vi "Datasheet Retrieve Table Data.vi"(4 "Datasheets to Generate":T3[](array[typedef]), 5 "Grouped Results":cluster{"Result Group":T6[]}[](array[cluster]), 6 "Paths":T5[](array[typedef]), 7 "Generator Settings":T2={"Wait? (t)"=TRUE, "ClientPrint? (f)"=FALSE, "Client (\"\")"="", "joinPDF"=FALSE, "Sort Method"=enum."Item", "Export Row (-1=all)"=-1, "Preview"=FALSE, "Estimate Time"=FALSE, "username"="", "jobid"=""}, 8 "error in (no error)":errorcluster, 9 "Parameters":T4, 10 "Template Record":T7, 11 "Connection Refnum":T1) -> (0 "error out":errorcluster, 1 "Datasheets to Generate":T3[](array[typedef]), 2 "Paths":T5[](array[typedef]), 3 "Connection Refnum":T1)   [LabVIEW 2011]
uses:
  database/Templates/Template Record.ctl
  Addons/internet/utils/keyedarr.llb/Keyed Array.ctl
  www/cgi-bin/_cgi-lib/TDM_INDEX Record.ctl
  SI.LIB/ODBC/SQL Controls/Connection Refnum.ctl
  Datasheet Report Info.ctl
  lib/datasheet script data.ctl
  Datasheet Generator Settings.ctl
  Addons/internet/utils/strutil.llb/Case Matching.ctl
  Column Data.ctl
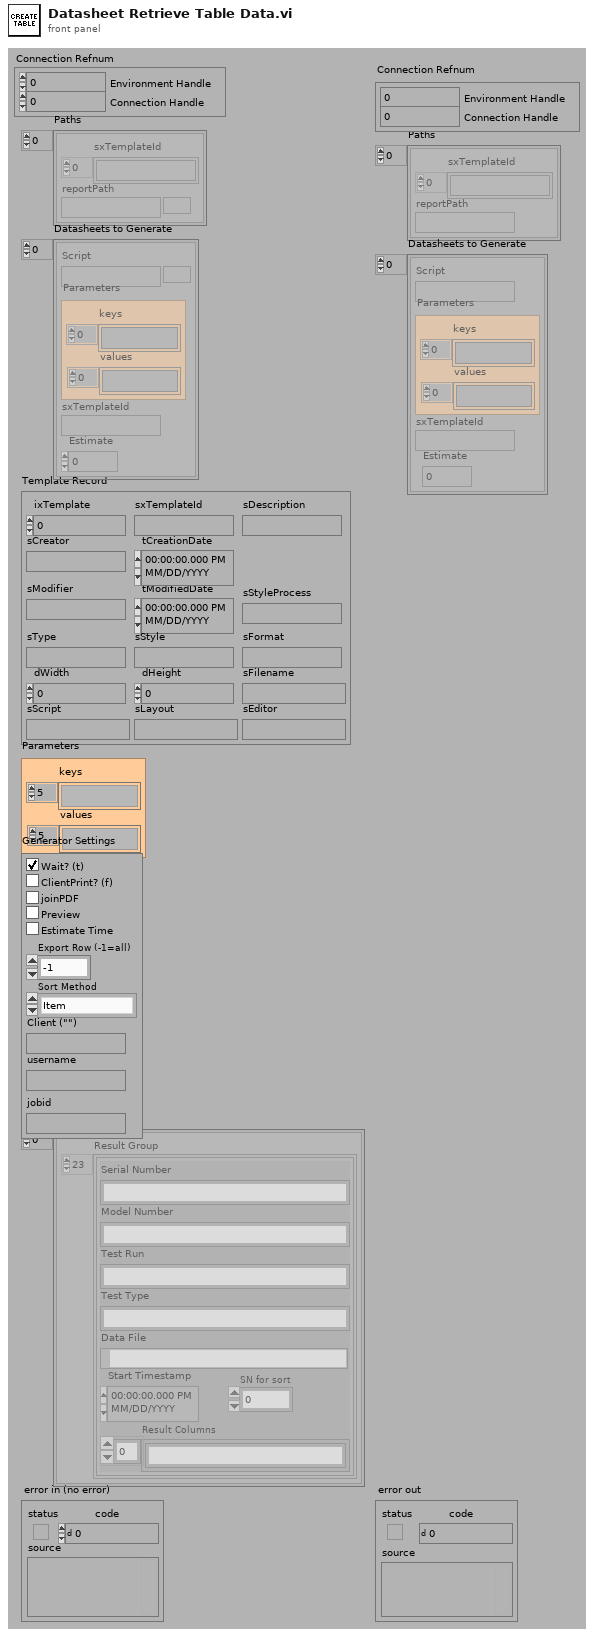
[diagram p1: front panel]
types:
  T1 = typedef "Connection Refnum.ctl" = cluster{"Environment Handle":i32, "Connection Handle":i32}
  T2 = typedef "DATASHEET Generator Settings.ctl" = cluster{"Wait? (t)":bool, "ClientPrint? (f)":bool, "Client (\"\")":string, "joinPDF":bool, "Sort Method":enum16{"Item", "Template", "No Sort"}, "Export Row (-1=all)":i32, "Preview":bool, "Estimate Time":bool, "username":string, "jobid":string}
  T3 = typedef "datasheet script data.ctl" = cluster{"Script":path, "Parameters":T4, "sxTemplateId":string, "Estimate":i32}
  T4 = typedef "Keyed Array.ctl" = cluster{"keys":string[], "values":string[]}
  T5 = typedef "Datasheet Report Info.ctl" = cluster{"sxTemplateId":string[], "reportPath":path}
  T6 = typedef "TDM_INDEX Record.ctl" = cluster{"Model Number":string, "SN for sort":i32, "Test Type":string, "Test Run":string, "Serial Number":string, "Start Timestamp":timestamp, "Data File":path, "Result Columns":string[]}
  T7 = typedef "Template Record.ctl" = cluster{"ixTemplate":i32, "sxTemplateId":string, "sDescription":string, "sCreator":string, "tCreationDate":timestamp, "sModifier":string, "tModifiedDate":timestamp, "sType":string, "sStyle":string, "sFormat":string, "dWidth":dbl, "dHeight":dbl, "sFilename":string, "sScript":string, "sLayout":string, "sEditor":string, "sStyleProcess":string}
  T8 = typedef "Case Matching.ctl" = enum16{"a != A", "a == A", "system"}
  T9 = typedef "Column Data.ctl" = cluster{"Run Select (Field=value)":string, "Type":string, "Parameters (comma list)":string, "Column Label":string}
  T10 = typedef "Field Record.ctl" = cluster{"ixField":i32, "iSequenceOrder":i32, "sxFieldId":string, "sxSequenceId":string, "sDisplayName":string, "sValue":string, "sUnits":string, "nDataType":T11, "nNextItem":T12, "fSystem":bool, "fSystemValue":bool, "fRequired":bool, "fSetAtTest":bool, "fTestField":bool, "fDeleted":bool, "fIndexed":bool, "fFreeList":bool}
  T11 = typedef "Field DataTypes.ctl" = enum32{"text", "numeric", "list", "timestamp", "boolean"}
  T12 = typedef "Field NextItem.ctl" = enum32{"Reset", "Retain", "Auto-Increment"}
  T13 = typedef "TDMS Model Number.ctl" = cluster{"Model Number":string, "Serial Number Tree Data":T14[]}
  T14 = typedef "TDMS Serial Number.ctl" = cluster{"Serial Number":string, "TDM Files":T15[]}
  T15 = typedef "TDMS File.ctl" = cluster{"File Path":path, "Run Data":T16[], "Serial Number":string, "Model Number":string, "Test Type":string}
  T16 = typedef "TDMS Run.ctl" = cluster{"Channel Data":T17[], "Custom Fields":T10[], "Run ID":string}
  T17 = typedef "TDMS Channel (Sxx).ctl" = cluster{"Channel Name":string, "Waveform":dbl[], "Unit":string, "List value":string}
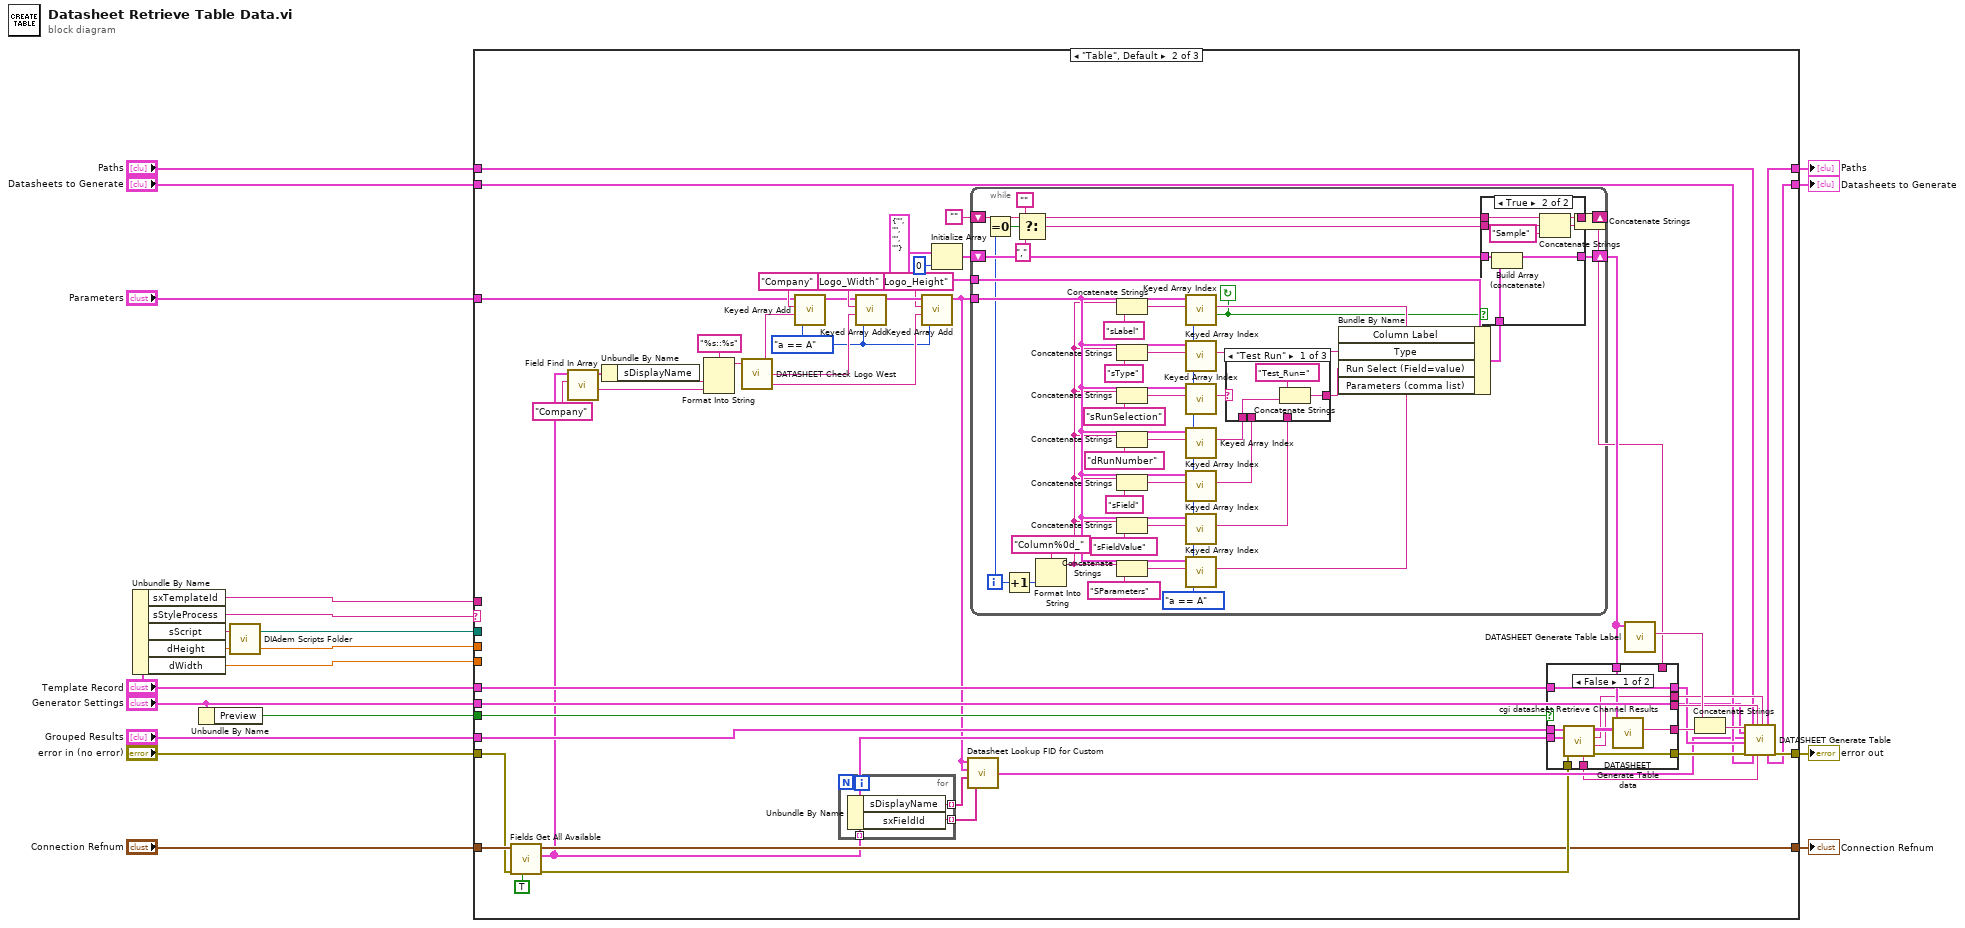
[diagram p0: block diagram]
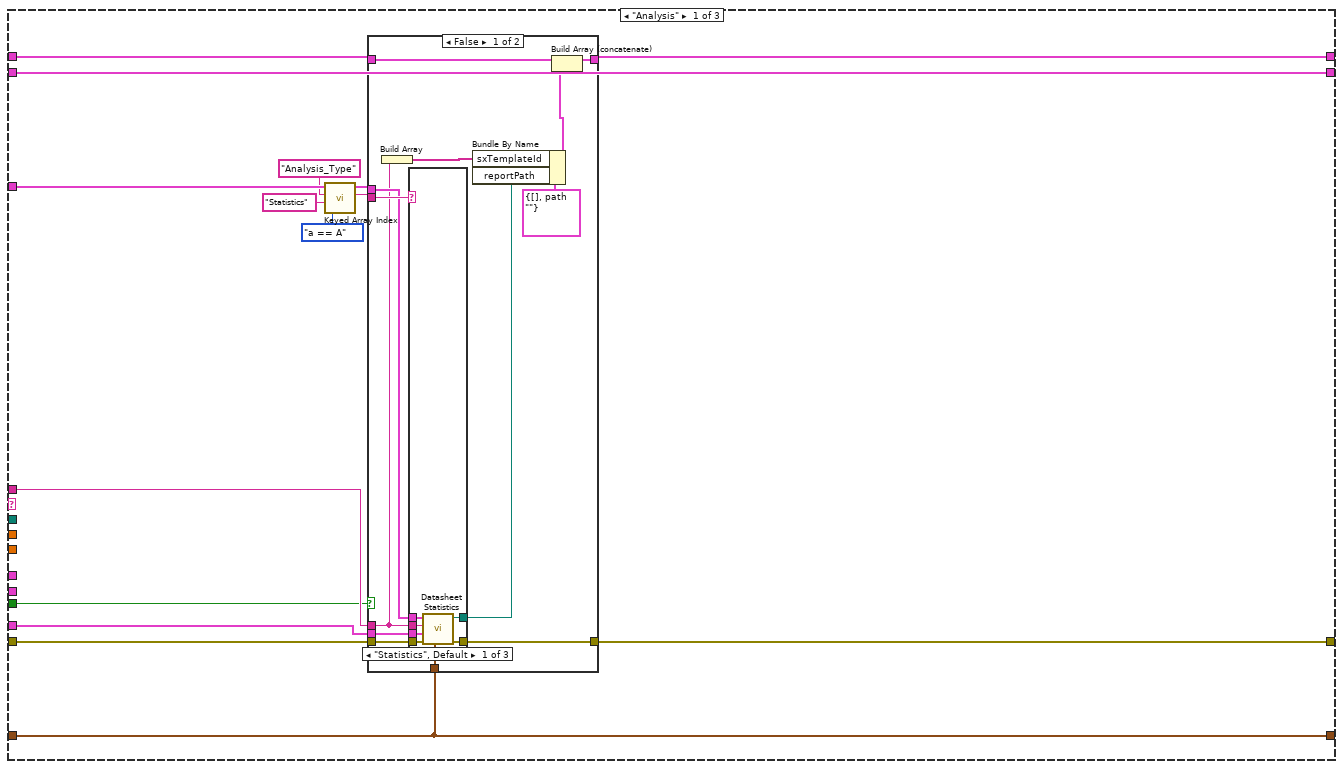
[diagram p2: hidden frame]
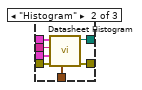
[diagram p3: hidden frame]
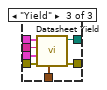
[diagram p4: hidden frame]
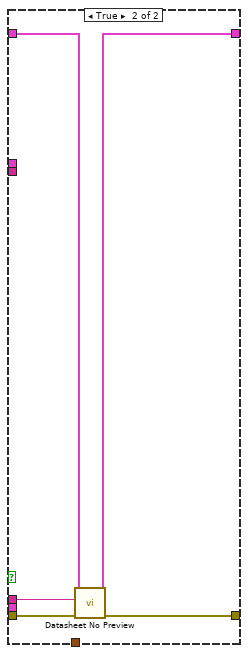
[diagram p5: hidden frame]
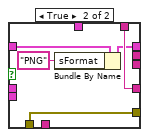
[diagram p6: hidden frame]
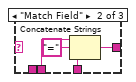
[diagram p7: hidden frame]
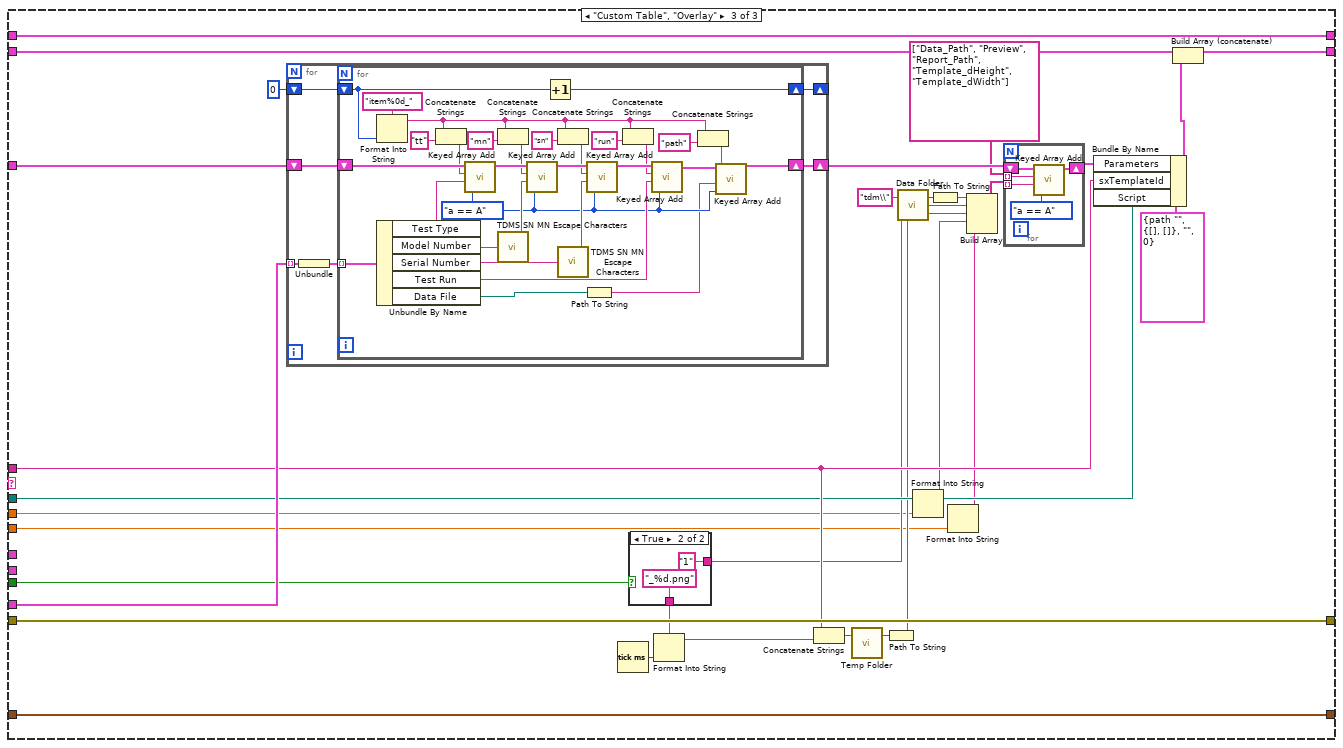
[diagram p10: hidden frame]
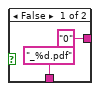
[diagram p11: hidden frame]
diagram:
  n1 = Unbundle By Name("Template Record") -> ("sxTemplateId"=w15:string, "sStyleProcess"=w19:string, "sScript"=w12:string, "dHeight"=w3:dbl, "dWidth"=w2:dbl)
  n2 = Unbundle By Name("Generator Settings") -> ("Preview"=w6:bool)
  n3 = call "DIAdem Scripts Folder.vi"("Relative Path (\"\" - Folder)"=w12) -> ("Scripts Folder"=w11:path)  [unwired: 2 out]
  n4 = case shown="\"Table\", Default" w19 {
    tunnel: "Parameters" -> [w31 w75 w230]
    tunnel: "error in (no error)" -> [w34 w99 w224]
    tunnel: [w32 w118 w224] -> w18
    tunnel: "Template Record" -> [_ w109 _]
    tunnel: "Grouped Results" -> [w33 w96 w229]
    tunnel: w15 -> [w24 _ w212]
    tunnel: "Connection Refnum" -> [w23 w100 w218]
    tunnel: w6 -> [w22 w103 w225]
    tunnel: w11 -> [_ _ w211]
    tunnel: "Paths" -> [w27 w107 w223]
    tunnel: [w26 w106 w223] -> w9
    tunnel: "Datasheets to Generate" -> [w25 w105 w222]
    tunnel: [w25 w104 w221] -> w7
    tunnel: "Generator Settings" -> [_ w97 _]
    tunnel: [w23 w95 w218] -> w4
    tunnel: w3 -> [_ _ w201]
    tunnel: w2 -> [_ _ w200]
    frame "Analysis" {
      n5 = call "Keyed Array Index.vi"("case matching (sensitive)"=Case_Matching."a == A", "default value"="Statistics", "key"="Analysis_Type", "array in"=w31) -> ("value"=w29:string, "duplicate array"=w21:T4)  [unwired: 2 out]
      n6 = case shown="False" w22 {
        tunnel: w34 -> [w47 w71]
        tunnel: w33 -> [w46 _]
        tunnel: [w45 w70] -> w32
        tunnel: w24 -> [w36 w69]
        tunnel: w23 -> [w44 _]
        tunnel: w29 -> [w43 _]
        tunnel: w27 -> [w42 w73]
        tunnel: [w41 w72] -> w26
        tunnel: w21 -> [w37 _]
        frame False {
          n7 = Build Array(w36) -> (w38:string[])
          n8 = case shown="\"Statistics\", Default" w43 {
            tunnel: w47 -> [w54 w61 w68]
            tunnel: w46 -> [w53 w60 w67]
            tunnel: w37 -> [w52 w59 w66]
            tunnel: [w51 w58 w65] -> w39
            tunnel: [w50 w57 w64] -> w45
            tunnel: w36 -> [w49 w56 w63]
            tunnel: w44 -> [w48 w55 w62]
            frame "Statistics", Default {
              n9 = call "Datasheet Statistics.vi"("Connection Refnum"=w48, "error in (no error)"=w54, "Grouped Results"=w53, "sxTemplateId"=w49, "Parameters"=w52) -> ("error out"=w50:errorcluster, "report"=w51:path)  [unwired: 5 in]
            }
            frame "Histogram" {
              n10 = call "Datasheet Histogram.vi"("Connection Refnum"=w55, "error in (no error)"=w61, "Grouped Results"=w60, "sxTemplateId"=w56, "Parameters"=w59) -> ("error out"=w57:errorcluster, "report"=w58:path)  [unwired: 5 in]
            }
            frame "Yield" {
              n11 = call "Datasheet Yield.vi"("Connection Refnum"=w62, "error in (no error)"=w68, "Grouped Results"=w67, "sxTemplateId"=w63, "Parameters"=w66) -> ("error out"=w64:errorcluster, "report"=w65:path)  [unwired: 5 in]
            }
          }
          n12 = Bundle By Name(cluster=T5 {"sxTemplateId"=[], "reportPath"=path ""} ("report"), "sxTemplateId"=w38, "reportPath"=w39) -> (w40:T5)
          n13 = Build Array (concatenate)(w42, w40) -> (w41:T5[])
        }
        frame True {
          n14 = call "Datasheet No Preview.vi"("error in"=w71, "sxTemplateId"=w69, "Paths"=w73) -> ("error out"=w70:errorcluster, "Array"=w72:T5[])  [unwired: 7 out]
        }
      }
    }
    frame "Table", Default {
      w87 = Case_Matching."a == A" ("case matching (sensitive)")
      w122 = T9 {"Run Select (Field=value)"="", "Type"="", "Parameters (comma list)"="", "Column Label"=""} ("Column Data")
      n15 = call "Fields Get All Available.vi"("Combine All? (f)"=TRUE, "error in (no error)"=w99, "Connection Refnum"=w100) -> ("error out"=w98:errorcluster, "System or ALL Combined Fields"=w79:T10[], "Connection Refnum"=w95:T1)  [unwired: 2 in, 4 out]
      n16 = call "Field Find In Array.vi"("FieldID or Display Name(\"\")"="Company" ("format string"), "Field Array"=w79) -> ("sValue"=w78:string, "Field"=w77:T10)  [unwired: 1 in, 7 out]
      n17 = Unbundle By Name(w77) -> ("sDisplayName"=w76:string)
      n18 = Format Into String(format string="%s::%s", w76, w78) -> (resulting string=w81:string)  [unwired: 2 in, 1 out]
      n19 = call "DATASHEET Check Logo West.vi"("Company_ID_Txt"=w81) -> ("Insertion Height"=w91:string, "Insertion Width"=w90:string, "Company_ID_Txt"=w88:string)  [unwired: 2 out]
      n20 = call "Keyed Array Add.vi"("case matching (sensitive)"=w87, "value"=w88, "key"="Company" ("format string"), "array in"=w75) -> ("array out"=w83:T4)  [unwired: 3 out]
      n21 = for {
        tunnel: w79 -> [w127] mode=indexing
        tunnel: [w126] -> w94 mode=indexing
        tunnel: [w125] -> w93 mode=indexing
        n22 = Unbundle By Name(w127) -> ("sDisplayName"=w126:string, "sxFieldId"=w125:string)
      }
      n23 = call "Keyed Array Add.vi"("case matching (sensitive)"=w87, "value"=w90, "key"="Logo_Width" ("format string"), "array in"=w83) -> ("array out"=w86:T4)  [unwired: 3 out]
      n24 = call "Keyed Array Add.vi"("case matching (sensitive)"=w87, "value"=w91, "key"="Logo_Height" ("format string"), "array in"=w86) -> ("array out"=w74:T4)  [unwired: 3 out]
      n25 = Initialize Array(w122, 0 ("dimension size")) -> (w124:T9[])
      n26 = call "Datasheet Lookup FID for Custom.vi"("sxFieldId"=w93, "Display Names"=w94, "Modified Report Parameters"=w74, "Original Parameters"=w74) -> ("Report Parameters"=w102:T4)
      n27 = while {
        tunnel: w74 -> [w154]
        shift-right: [w180] -> w121
        shift-left: w124 -> [w177]
        tunnel: w122 -> [w178]
        shift-right: [w164] -> w114
        shift-left: "" -> [w163]
        i -> [w144]
        stop <- w165 continue-if-true
        w153 = Case_Matching."a == A" ("case matching (sensitive)")
        n28 = Equal To 0?(x=w144) -> (x = 0?=w160:bool)
        n29 = Increment(x=w144) -> (x+1=w182:i32)
        n30 = Select(t="", s=w160, f="," ("format string")) -> (s? t:f=w161:string)
        n31 = Format Into String(format string="Column%0d_", w182) -> (resulting string=w146:string)  [unwired: 2 in, 1 out]
        n32 = Concatenate Strings(w146, "sLabel" ("format string")) -> (w176:string)
        n33 = Concatenate Strings(w146, "sType" ("format string")) -> (w173:string)
        n34 = Concatenate Strings(w146, "sRunSelection" ("format string")) -> (w172:string)
        n35 = Concatenate Strings(w146, "dRunNumber" ("format string")) -> (w157:string)
        n36 = Concatenate Strings(w146, "sField" ("format string")) -> (w156:string)
        n37 = Concatenate Strings(w146, "sFieldValue" ("format string")) -> (w155:string)
        n38 = Concatenate Strings(w146, "SParameters" ("format string")) -> (w170:string)
        n39 = call "Keyed Array Index.vi"("case matching (sensitive)"=w153, "key"=w176, "array in"=w154) -> ("valid key"=w165:bool, "value"=w168:string)  [unwired: 1 in, 2 out]
        n40 = call "Keyed Array Index.vi"("case matching (sensitive)"=w153, "key"=w173, "array in"=w154) -> ("value"=w167:string)  [unwired: 1 in, 3 out]
        n41 = call "Keyed Array Index.vi"("case matching (sensitive)"=w153, "key"=w172, "array in"=w154) -> ("value"=w158:string)  [unwired: 1 in, 3 out]
        n42 = call "Keyed Array Index.vi"("case matching (sensitive)"=w153, "key"=w157, "array in"=w154) -> ("value"=w149:string)  [unwired: 1 in, 3 out]
        n43 = call "Keyed Array Index.vi"("case matching (sensitive)"=w153, "key"=w156, "array in"=w154) -> ("value"=w151:string)  [unwired: 1 in, 3 out]
        n44 = call "Keyed Array Index.vi"("case matching (sensitive)"=w153, "key"=w155, "array in"=w154) -> ("value"=w150:string)  [unwired: 1 in, 3 out]
        n45 = call "Keyed Array Index.vi"("case matching (sensitive)"=w153, "key"=w170, "array in"=w154) -> ("value"=w166:string)  [unwired: 1 in, 3 out]
        n46 = case shown="\"Test Run\"" w158 {
          selector: w158 -> [_ _ w190]
          tunnel: [w184 w188 w190] -> w152
          tunnel: w151 -> [_ w186 _]
          tunnel: w150 -> [_ w187 _]
          tunnel: w149 -> [w183 _ _]
          frame "Test Run" {
            n47 = Concatenate Strings("Test_Run=" ("format string"), w183) -> (w184:string)
          }
          frame "Match Field" {
            n48 = Concatenate Strings(w186, "=" ("format string"), w187) -> (w188:string)
          }
          frame "Most Recent", Default {
          }
        }
        n49 = Bundle By Name(cluster=w178, "Column Label"=w168, "Type"=w167, "Run Select (Field=value)"=w152, "Parameters (comma list)"=w166) -> (w179:T9)
        n50 = case shown="True" w165 {
          tunnel: [w192 w199] -> w180
          tunnel: w179 -> [_ w198]
          tunnel: w177 -> [w192 w197]
          tunnel: [w191 w196] -> w164
          tunnel: w163 -> [w191 w194]
          tunnel: w161 -> [_ w193]
          frame False {
          }
          frame True {
            n51 = Build Array (concatenate)(w197, w198) -> (w199:T9[])
            n52 = Concatenate Strings(w194, w193, "Sample" ("format string")) -> (w196:string)
          }
        }
      }
      n53 = Concatenate Strings(w114, "\n") -> (w113:string)
      n54 = case shown="False" w103 {
        tunnel: w121 -> [w138 _]
        tunnel: [w137 w143] -> w119
        tunnel: w96 -> [w136 _]
        tunnel: w98 -> [w135 w139]
        tunnel: [w134 w139] -> w116
        tunnel: w113 -> [_ w143]
        tunnel: [w132 _] -> w111
        tunnel: [w131 _] -> w110
        tunnel: w109 -> [w130 w142]
        tunnel: [w130 w141] -> w108
        tunnel: w79 -> [w129 _]
        tunnel: [w128 _] -> w92
        frame False {
          n55 = call "cgi datasheet Retrieve Channel Results.vi"("error in (no error)"=w135, "All Combined Fields"=w129, "Grouped Results"=w136) -> ("error out"=w134:errorcluster, "First Item Run"=w131:string, "First Item Path"=w132:string, "Data Tree"=w133:T13[][], "First Item Test Type"=w128:string)  [unwired: 4 in]
          n56 = call "DATASHEET Generate Table data.vi"("Data Tree"=w133, "Column Data"=w138) -> ("Comma rows"=w137:string)  [unwired: 1 in, 8 out]
        }
        frame True {
          n57 = Bundle By Name(cluster=w142, "sFormat"="PNG") -> (w141:T7)
        }
      }
      n58 = call "DATASHEET Generate Table Label.vi"("Column Data"=w121) -> ("Comma Label Row"=w120:string)  [unwired: 3 in, 7 out]
      n59 = Concatenate Strings(w120, w119) -> (w117:string)
      n60 = call "DATASHEET Generate Table.vi"("ASCII table"=w117, "Preview?"=w97, "Parameters"=w102, "Template Record"=w108, "error in (no error)"=w116, "Paths"=w107, "Datasheets to Generate"=w105, "First Item Run"=w110, "First Item Test Type"=w92, "First Item Path"=w111) -> ("Paths Out"=w106:T5[], "Datasheets to Generate Out"=w104:T3[], "error out"=w118:errorcluster)  [unwired: 7 out]
    }
    frame "Custom Table", "Overlay" {
      n61 = for {
        shift-right: [w243] -> w205
        shift-left: w230 -> [w244]
        tunnel: w229 -> [w245] mode=indexing
        shift-right: [w241] -> _
        shift-left: 0 -> [w242]
        n62 = Unbundle(w245) -> ("Result Group"=w240:T6[])
        n63 = for {
          tunnel: w240 -> [w275] mode=indexing
          shift-right: [w249] -> w243
          shift-left: w244 -> [w271]
          shift-right: [w260] -> w241
          shift-left: w242 -> [w261]
          w250 = Case_Matching."a == A" ("case matching (sensitive)")
          n64 = Format Into String(format string="item%0d_" ("key"), w261) -> (resulting string=w251:string)  [unwired: 2 in, 1 out]
          n65 = Unbundle By Name(w275) -> ("Test Type"=w270:string, "Model Number"=w257:string, "Serial Number"=w255:string, "Test Run"=w269:string, "Data File"=w247:path)
          n66 = Concatenate Strings(w251, "tt" ("key")) -> (w263:string)
          n67 = call "Keyed Array Add.vi"("case matching (sensitive)"=w250, "value"=w270, "key"=w263, "array in"=w271) -> ("array out"=w272:T4)  [unwired: 3 out]
          n68 = Concatenate Strings(w251, "mn" ("key")) -> (w259:string)
          n69 = call "TDMS SN MN Escape Characters.vi"("string"=w257) -> ("url-encoded string"=w256:string)
          n70 = call "Keyed Array Add.vi"("case matching (sensitive)"=w250, "value"=w256, "key"=w259, "array in"=w272) -> ("array out"=w274:T4)  [unwired: 3 out]
          n71 = Increment(x=w261) -> (x+1=w260:i32)
          n72 = Concatenate Strings(w251, "sn" ("key")) -> (w258:string)
          n73 = call "TDMS SN MN Escape Characters.vi"("string"=w255) -> ("url-encoded string"=w254:string)
          n74 = Path To String(path=w247) -> (string=w246:string)
          n75 = call "Keyed Array Add.vi"("case matching (sensitive)"=w250, "value"=w254, "key"=w258, "array in"=w274) -> ("array out"=w273:T4)  [unwired: 3 out]
          n76 = Concatenate Strings(w251, "run" ("key")) -> (w268:string)
          n77 = call "Keyed Array Add.vi"("case matching (sensitive)"=w250, "value"=w269, "key"=w268, "array in"=w273) -> ("array out"=w252:T4)  [unwired: 3 out]
          n78 = Concatenate Strings(w251, "path" ("string")) -> (w253:string)
          n79 = call "Keyed Array Add.vi"("case matching (sensitive)"=w250, "value"=w246, "key"=w253, "array in"=w252) -> ("array out"=w249:T4)  [unwired: 3 out]
        }
      }
      n80 = Tick Count (ms)() -> (millisecond timer value=w215:u32)
      n81 = case shown="True" w225 {
        tunnel: ["_%d.pdf" "_%d.png"] -> w213
        tunnel: ["0" ("format string") "1" ("format string")] -> w209
        frame False {
        }
        frame True {
        }
      }
      n82 = Format Into String(format string=w213, w215) -> (resulting string=w214:string)  [unwired: 2 in, 1 out]
      n83 = Concatenate Strings(w212, w214) -> (w216:string)
      n84 = call "Temp Folder.vi"("Relative Path (\"\")"=w216) -> ("Temp Folder"=w217:path)  [unwired: 2 in]
      n85 = Path To String(path=w217) -> (string=w208:string)
      n86 = call "Data Folder.vi"("Relative Path (\"\" - Folder)"="tdm\\") -> ("Data Folder"=w227:path)  [unwired: 2 in]
      n87 = Format Into String(w201) -> (resulting string=w207:string)  [unwired: 3 in, 1 out]
      n88 = Path To String(path=w227) -> (string=w210:string)
      n89 = Format Into String(w200) -> (resulting string=w206:string)  [unwired: 3 in, 1 out]
      n90 = Build Array(w210, w209, w208, w207, w206) -> (w202:string[])
      n91 = for {
        shift-right: [w233] -> w204
        shift-left: w205 -> [w234]
        tunnel: string[] ["Data_Path", "Preview", "Report_Path", "Template_dHeight", "Template_dWidth"] -> [w232] mode=indexing
        tunnel: w202 -> [w231] mode=indexing
        n92 = call "Keyed Array Add.vi"("case matching (sensitive)"=Case_Matching."a == A", "value"=w231, "key"=w232, "array in"=w234) -> ("array out"=w233:T4)  [unwired: 3 out]
      }
      n93 = Bundle By Name(cluster=T3 {"Script"=path "", "Parameters"={"keys"=[], "values"=[]}, "sxTemplateId"="", "Estimate"=0} ("Datasheet"), "Parameters"=w204, "sxTemplateId"=w212, "Script"=w211) -> (w220:T3)
      n94 = Build Array (concatenate)(w222, w220) -> (w221:T3[])
    }
  }
  "error out" <- w18
  "Paths" <- w9
  "Datasheets to Generate" <- w7
  "Connection Refnum" <- w4
